vi "Get Lvlibp Messages.vi"(8 "error in (no error)":errorcluster) -> (0 "error out":errorcluster, 1 "Classes Loaded":bool, 2 "Supports Data Access?":bool[](array[boolean]), 3 "Msg Paths":path[](array[path]))   [LabVIEW 2020, in "Sequencer.lvlib"]
doc: "Get paths to all messages in either the Folder Override folder or in the PPL folder.\nMessages are only recognized if their class name ends with msg.lvclass (not case sensitive).\nAll found messages are checked for the Data Access.vi. This VI will only be detected if it is placed in the same folder as the message class."
uses:
  Sequencer.lvlib
  PPL/HDH.ClassLoader.lvlibp/Sub/Ctl/Ctl_Front-load Scope.ctl
  PPL/HDH.ClassLoader.lvlibp
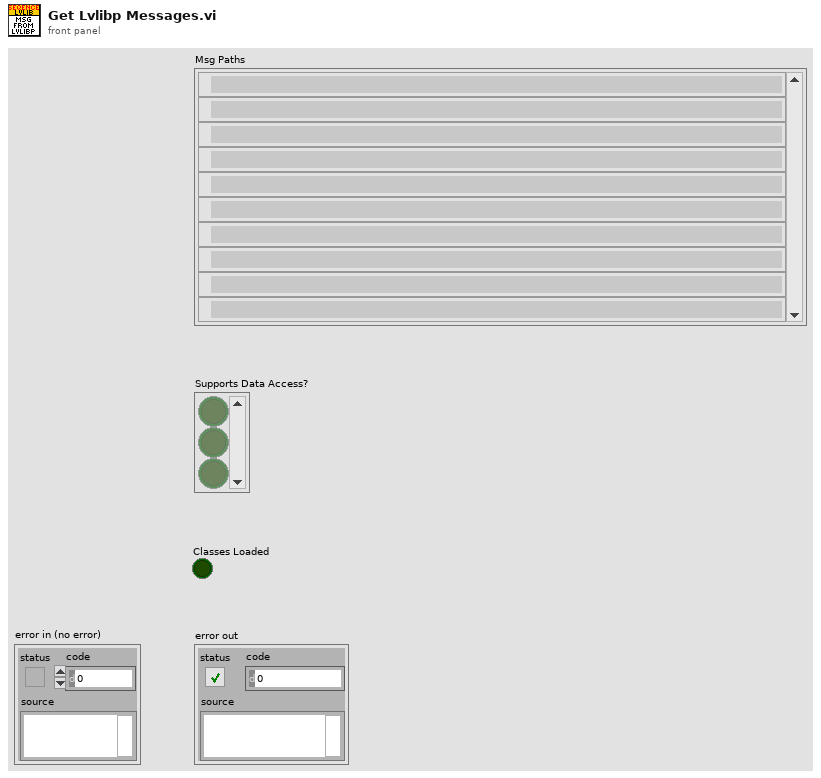
[diagram p1: front panel]
types:
  T1 = typedef "HDH.ClassLoader.lvlibp/Ctl_Front-load Scope.ctl" = enum16{"Paths", "Paths and Hierarchies", "All"}
  T2 = typedef "HDH.ClassLoader.lvlibp/Ctl_Member Map.ctl" = map{string, T3}
  T3 = typedef "HDH.ClassLoader.lvlibp/HDH.ClassLoader_Member VI Info.ctl" = cluster{"qualified name":string, "path":path, "access scope":enum32{"invalid scope", "public", "private", "protected", "community"}, "is dynamic dispatch":bool}
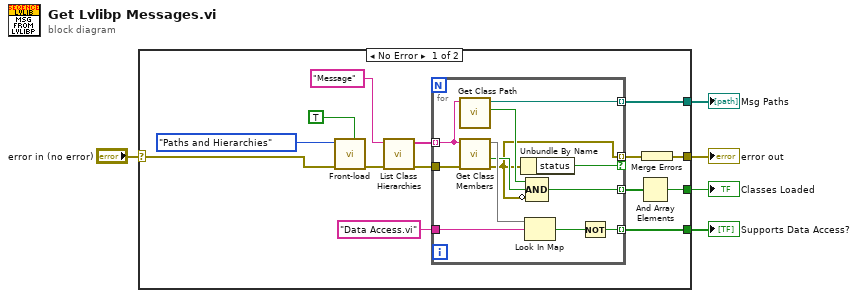
[diagram p0: block diagram]
diagram:
  n1 = case shown="No Error" "error in (no error)" {
    selector: "error in (no error)" -> [w16 w32]
    tunnel: [w19 _] -> w5
    tunnel: [w18 _] -> w4
    tunnel: [w17 w32] -> w2
    tunnel: [w15 _] -> w1
    frame No Error {
      n2 = call "Front-load.vi"("Show UI?(F)"=TRUE, "error in (no error)"=w16, "Scope(Paths)"=Ctl_Front-load_Scope."Paths and Hierarchies") -> ("error out"=w12:errorcluster)  [unwired: 7 in, 1 out]
      n3 = call "List Class Hierarchies.vi"("error in (no error)"=w12, "Hierarchy Filter(empty=all)"="Message") -> ("error out"=w9:errorcluster, "Classes found"=w10:string[])  [unwired: 6 in, 2 out]
      n4 = for {
        tunnel: w10 -> [w26] mode=indexing
        tunnel: w9 -> [w31]
        tunnel: "Data Access.vi" ("name or relative path") -> [w29]
        tunnel: [w27] -> w19 mode=indexing
        tunnel: [w21] -> w7 mode=indexing if=w25
        tunnel: [w24] -> w18 mode=indexing
        tunnel: [w20] -> w6 mode=indexing
        n5 = call "Get Class Path.vi"("Base Class Name"=w26) -> ("Success?"=w23:bool, "Path"=w24:path)  [unwired: 9 in]
        n6 = call "Get Class Members.vi"("error in (no error)"=w31, "Base Class Name"=w26) -> ("error out"=w21:errorcluster, "Success?"=w22:bool, "Member Map"=w30:T2)  [unwired: 7 in]
        n7 = Unbundle By Name(w21) -> ("status"=w25:bool)
        n8 = Look In Map(map=w30, key=w29) -> (key not found?=w28:bool)  [unwired: 1 in, 1 out]
        n9 = Compound Arithmetic op=AND(w23, w22, invert w21) -> (w20:bool)
        n10 = Not(x=w28) -> (.not. x?=w27:bool)
      }
      n11 = And Array Elements(Boolean array=w6) -> (logical AND=w15:bool)
      n12 = Merge Errors(w7) -> (w17:errorcluster)
    }
    frame Error {
    }
  }
  "Supports Data Access?" <- w5
  "Msg Paths" <- w4
  "error out" <- w2
  "Classes Loaded" <- w1
